vi "Initialize.vi"(8 "error in (no error)":errorcluster, 9 "Reset (True)":bool=TRUE, 10 "ID Query (True)":bool=TRUE, 11 "VISA resource name":refnum<visa-resource-name>) -> (0 "error out":errorcluster, 3 "VISA resource name out":refnum<visa-resource-name>)   [LabVIEW 2025, in "Keithley DMM7510.lvlib"]
doc: "Establishes communication with the instrument and optionally performs an instrument identification query and/or an instrument reset. It also places the instrument in a default state needed for other instrument driver operations. Therefore, call this VI before calling other instrument driver VIs for this instrument. Generally, you need to call the Initialize VI only once at the beginning of an application."
uses:
  Keithley DMM7510.lvlib
panel:
  # "(c) 2014 Keithley.  ALL RIGHTS RESERVED."
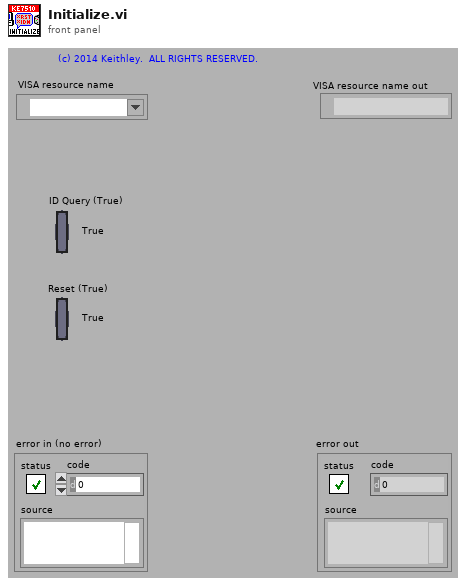
[diagram p1: front panel]
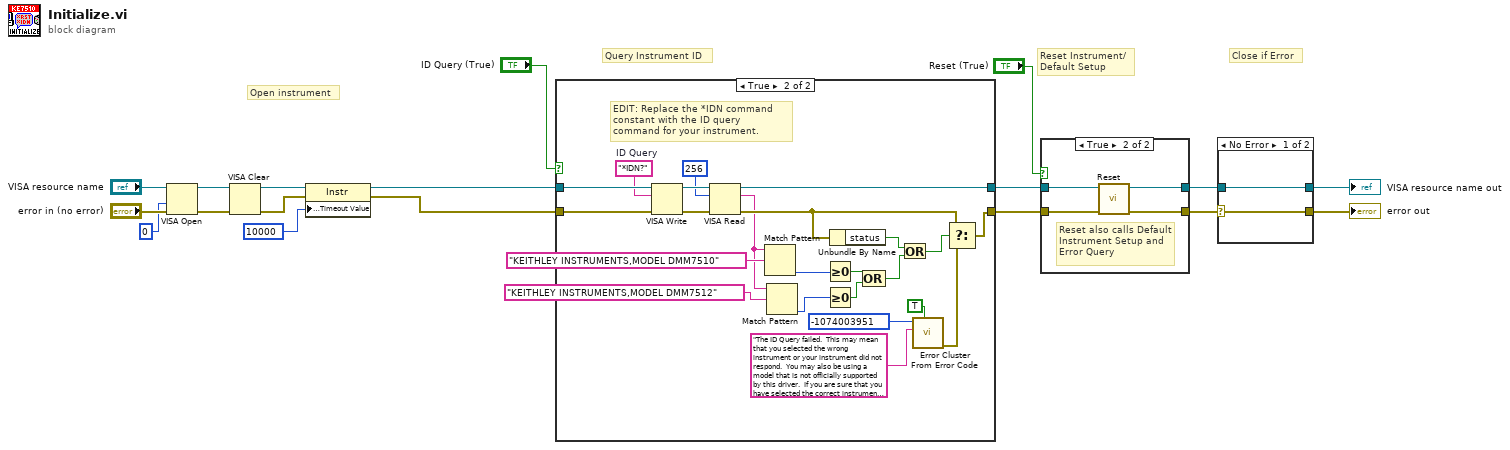
[diagram p0: block diagram]
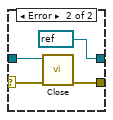
[diagram p2: hidden frame]
diagram:
  # "Close if Error"
  # "Query Instrument ID"
  # "Reset Instrument/\nDefault Setup"
  # "Open instrument"
  n1 = VISA Open(access mode=u32 0, error in (no error)="error in (no error)", VISA resource name="VISA resource name") -> (VISA resource name=w10:refnum<visa-resource-name>, error out=w9:errorcluster)  [unwired: 2 in]
  n2 = VISA Clear(VISA resource name=w10, error in (no error)=w9) -> (VISA resource name out=w8:refnum<visa-resource-name>, error out=w7:errorcluster)
  n3 = property class="Instr"(reference=w8, error in=w7, "General Settings:Timeout Value"=u32 10000) -> (reference out=w2:refnum<visa-resource-name>, error out=w1:errorcluster)
  n4 = case shown="True" "ID Query (True)" {
    tunnel: [w19 w43] -> w17
    tunnel: [w20 w40] -> w18
    tunnel: w2 -> [w20 w41]
    tunnel: w1 -> [w19 w42]
    frame False {
    }
    frame True {
      w35 = "*IDN?"  # ID Query
      # "EDIT: Replace the *IDN command\nconstant with the ID query\ncommand for your instrument."
      n5 = VISA Write(VISA resource name=w41, write buffer=w35, error in (no error)=w42) -> (VISA resource name out=w39:refnum<visa-resource-name>, error out=w38:errorcluster)  [unwired: 1 out]
      n6 = VISA Read(VISA resource name=w39, byte count=u32 256, error in (no error)=w38) -> (VISA resource name out=w40:refnum<visa-resource-name>, read buffer=w26:string, error out=w29:errorcluster)  [unwired: 1 out]
      n7 = Match Pattern(string=w26, regular expression="KEITHLEY INSTRUMENTS,MODEL DMM7510") -> (offset past match=w30:i32)  [unwired: 1 in, 3 out]
      n8 = Match Pattern(string=w26, regular expression="KEITHLEY INSTRUMENTS,MODEL DMM7512") -> (offset past match=w24:i32)  [unwired: 1 in, 3 out]
      n9 = Greater Or Equal To 0?(x=w30) -> (x >= 0?=w23:bool)
      n10 = Greater Or Equal To 0?(x=w24) -> (x >= 0?=w22:bool)
      n11 = Unbundle By Name(w29) -> ("status"=w28:bool)
      n12 = Compound Arithmetic op=OR(w23, w22) -> (w21:bool)
      n13 = Or(x=w28, y=w21) -> (x .or. y?=w27:bool)
      n14 = call <vilib>:"Error Cluster From Error Code.vi"("show call chain? (False)"=TRUE, "error message (\"\")"="The ID Query failed.  This may mean that you selected the wrong instrument or your instrument did not respond.  You may also be using a model that is not officially supported by this driver.  If you are sure that you have selected the correct instrument and it is responding, try disabling the ID Query." ("Source (VI Name)"), "error code (0)"=-1074003951 ("Code")) -> ("error out"=w34:errorcluster)  [unwired: 6 in]
      n15 = Select(t=w29, s=w27, f=w34) -> (s? t:f=w43:errorcluster)
    }
  }
  n16 = case shown="True" "Reset (True)" {
    tunnel: w17 -> [w44 w46]
    tunnel: [w44 w49] -> w3
    tunnel: w18 -> [w45 w47]
    tunnel: [w45 w48] -> w4
    frame False {
    }
    frame True {
      # "Reset also calls Default Instrument Setup and Error Query"
      n17 = call "Reset.vi"("error in (no error)"=w46, "VISA resource name"=w47) -> ("error out"=w49:errorcluster, "VISA resource name out"=w48:refnum<visa-resource-name>)  [unwired: 8 in]
    }
  }
  n18 = case shown="No Error" w3 {
    selector: w3 -> [w50 w53]
    tunnel: w4 -> [w51 w54]
    tunnel: [w51 refnum<visa-resource-name> refnum ("VISA resource name out")] -> w6
    tunnel: [w50 w55] -> w5
    frame No Error {
    }
    frame Error {
      n19 = call "Close.vi"("error in (no error)"=w53, "VISA resource name"=w54) -> ("error out"=w55:errorcluster)  [unwired: 9 in]
    }
  }
  "VISA resource name out" <- w6
  "error out" <- w5
